vi "Read Image Metadata FIFO.vi"(0 "fpga inteface in":refnum<k20>, 5 "display channel number":i32, 7 "number of images":u32, 11 "error in (no error)":errorcluster) -> (4 "fpga interface out":refnum<k20>, 6 "image metadata":T1[](array[typedef]), 8 "images remaining":u32, 15 "error out":errorcluster)   [LabVIEW 2023, in "GettingStarted_Common_148X_Host.lvlib"]
uses:
  GettingStarted_Common_148X_Host.lvlib
  FPGA/Common/Types/Image Metadata.ctl
  <instrlib>/FlexRIO/CSI-2/v2/Common/Types/LLP Data Type.ctl
  Types/148x_Common_FPGA_Reference.ctl
  <vilib>/rvi/errors/niLvFpgaAdjustHostInterfaceError.vi
  <instrlib>/_niInstr/Data Formatting/v1/FPGA/Private/Convert/U64 array to Boolean Array.vi
  <vilib>/rvi/interface/nirviMethod/nirviMethod.xnode
  <vilib>/FPGAPlugInAG/Dynamic/niLvFpga_ReadFifo_Dynamic.vi
  <vilib>/rvi/errors/niLvFpgaMergeErrorWithErrorCode.vi
  <instrlib>/_niInstr/Data Formatting/v1/FPGA/niInstr Data Formatting v1 FPGA.lvlib
  <instrlib>/FlexRIO/CSI-2/v2/Common/NI CSI-2 API Common v2.lvlib
  FPGA/Common/GettingStarted_Common_148X_FPGA.lvlib
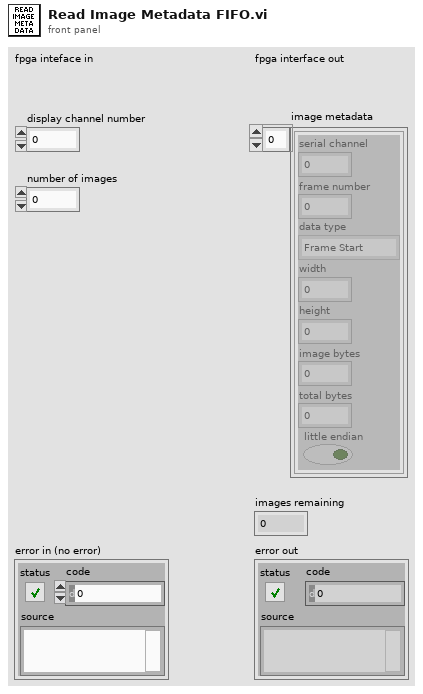
[diagram p1: front panel]
types:
  T1 = typedef "GettingStarted_Common_148X_FPGA.lvlib/Image Metadata.ctl" = cluster{"serial channel":fxp<+,3,3>, "frame number":u16, "data type":T2, "width":u16, "height":u16, "image bytes":u32, "total bytes":u32, "little endian":bool}
  T2 = typedef "NI CSI-2 API Common v2.lvlib/LLP Data Type.ctl" = enum8{"Frame Start", "Frame End", "Line Start", "Line End", "End of Transmission", "Reserved 0", "Reserved 1", "Reserved 2", "Generic Short Packet 1", "Generic Short Packet 2", "Generic Short Packet 3", "Generic Short Packet 4", "Generic Short Packet 5", "Generic Short Packet 6", "Generic Short Packet 7", "Generic Short Packet 8", "Null", "Blanking Data", "Embedded 8-bit non Image Data", "Generic Long Packet 1", "Generic Long Packet 2", "Generic Long Packet 3", "Generic Long Packet 4", "Reserved 3", "YUV420 8-bit", "YUV420 10-bit", "Legacy YUV420 8-bit", "Reserved 4", "YUV420 8-bit Chroma Shifted", "YUV420 10-bit Chroma Shifted", "YUV422 8-bit", "YUV422 10-bit", "RGB444", "RGB555", "RGB565", "RGB666", "RGB888", "Reserved 5", "Reserved 6", "RAW 24", "RAW 6", "RAW 7", "RAW 8", "RAW 10", "RAW 12", "RAW 14", "RAW 16", "RAW 20", "User Defined 8-bit Data 1", "User Defined 8-bit Data 2", "User Defined 8-bit Data 3", "User Defined 8-bit Data 4", "User Defined 8-bit Data 5", "User Defined 8-bit Data 6", "User Defined 8-bit Data 7", "User Defined 8-bit Data 8", "USL Command", "Reserved 7", "Reserved 8", "Reserved 9", "Reserved 10", "Reserved 11", "Reserved 12", "LRTE EPD Spacer"}
  T3 = typedef "GettingStarted_Common_148X_Host.lvlib/148x_Common_FPGA_Reference.ctl" = refnum<k20>
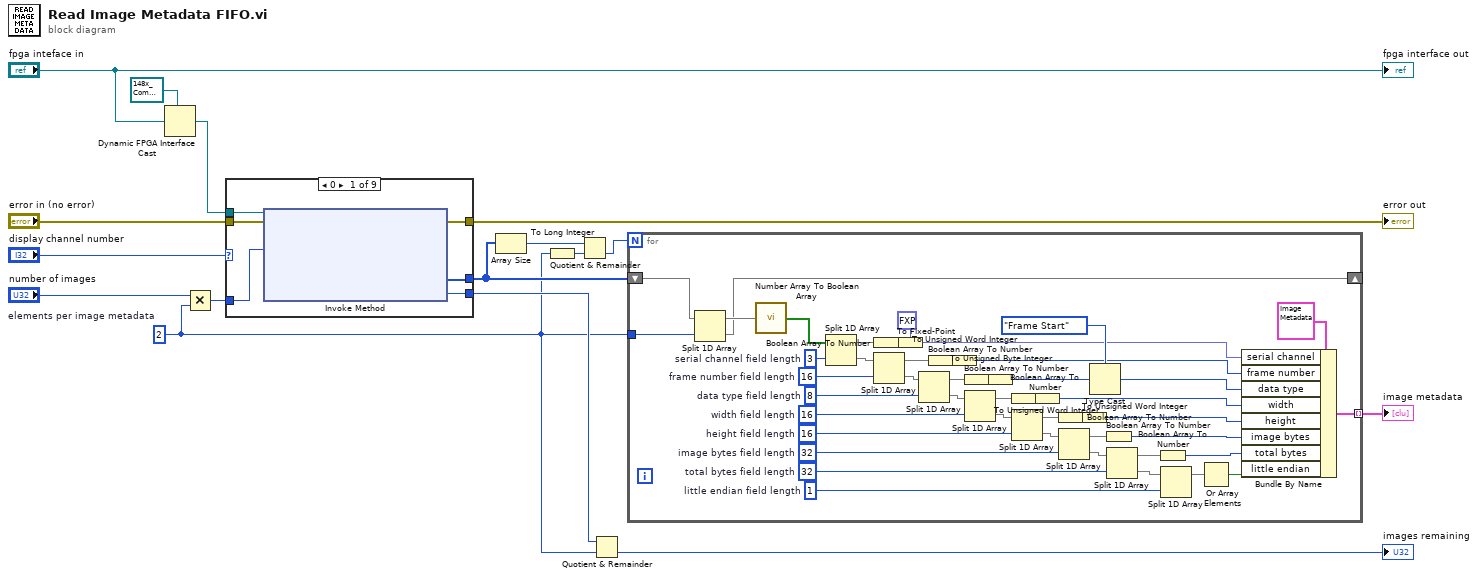
[diagram p0: block diagram]
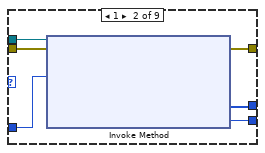
[diagram p2: hidden frame]
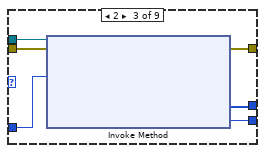
[diagram p3: hidden frame]
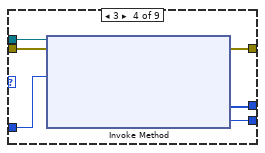
[diagram p4: hidden frame]
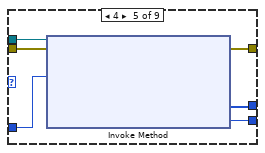
[diagram p5: hidden frame]
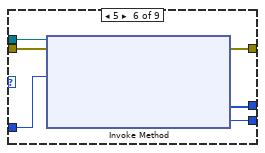
[diagram p6: hidden frame]
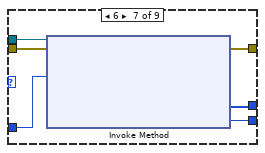
[diagram p7: hidden frame]
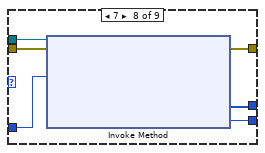
[diagram p8: hidden frame]
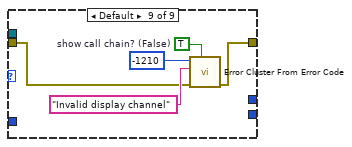
[diagram p9: hidden frame]
diagram:
  w3 = u32 2  # elements per image metadata
  n1 = Dynamic FPGA Interface Cast(Session In=T3 refnum ("FPGA VI Reference Out"), Type="fpga inteface in") -> (Session Out=w14:T3)
  n2 = Multiply(x="number of images", y=w3) -> (x*y=w9:u32)
  n3 = case shown="0" "display channel number" {
    tunnel: "error in (no error)" -> [w22 w28 w34 w40 w46 w52 w58 w64 w66]
    tunnel: w14 -> [w21 w27 w33 w39 w45 w51 w57 w63 _]
    tunnel: [w20 w26 w32 w38 w44 w50 w56 w62 w65] -> w10
    tunnel: w9 -> [w19 w25 w31 w37 w43 w49 w55 w61 _]
    tunnel: [w18 w24 w30 w36 w42 w48 w54 w60 _] -> w4
    tunnel: [w17 w23 w29 w35 w41 w47 w53 w59 _] -> w16
    frame 0 {
      n4 = xnode "Invoke Method"("FPGA VI Reference In"=w21, "error in"=w22, "Number of Elements"=w19) -> ("error out"=w20:errorcluster, "Data"=w18:u64[], "Elements Remaining"=w17:u32)  [unwired: 1 in, 1 out]
    }
    frame 1 {
      n5 = xnode "Invoke Method"("FPGA VI Reference In"=w27, "error in"=w28, "Number of Elements"=w25) -> ("error out"=w26:errorcluster, "Data"=w24:u64[], "Elements Remaining"=w23:u32)  [unwired: 1 in, 1 out]
    }
    frame 2 {
      n6 = xnode "Invoke Method"("FPGA VI Reference In"=w33, "error in"=w34, "Number of Elements"=w31) -> ("error out"=w32:errorcluster, "Data"=w30:u64[], "Elements Remaining"=w29:u32)  [unwired: 1 in, 1 out]
    }
    frame 3 {
      n7 = xnode "Invoke Method"("FPGA VI Reference In"=w39, "error in"=w40, "Number of Elements"=w37) -> ("error out"=w38:errorcluster, "Data"=w36:u64[], "Elements Remaining"=w35:u32)  [unwired: 1 in, 1 out]
    }
    frame 4 {
      n8 = xnode "Invoke Method"("FPGA VI Reference In"=w45, "error in"=w46, "Number of Elements"=w43) -> ("error out"=w44:errorcluster, "Data"=w42:u64[], "Elements Remaining"=w41:u32)  [unwired: 1 in, 1 out]
    }
    frame 5 {
      n9 = xnode "Invoke Method"("FPGA VI Reference In"=w51, "error in"=w52, "Number of Elements"=w49) -> ("error out"=w50:errorcluster, "Data"=w48:u64[], "Elements Remaining"=w47:u32)  [unwired: 1 in, 1 out]
    }
    frame 6 {
      n10 = xnode "Invoke Method"("FPGA VI Reference In"=w57, "error in"=w58, "Number of Elements"=w55) -> ("error out"=w56:errorcluster, "Data"=w54:u64[], "Elements Remaining"=w53:u32)  [unwired: 1 in, 1 out]
    }
    frame 7 {
      n11 = xnode "Invoke Method"("FPGA VI Reference In"=w63, "error in"=w64, "Number of Elements"=w61) -> ("error out"=w62:errorcluster, "Data"=w60:u64[], "Elements Remaining"=w59:u32)  [unwired: 1 in, 1 out]
    }
    frame Default {
      w67 = TRUE  # show call chain? (False)
      n12 = call <vilib>:"Error Cluster From Error Code.vi"("show call chain? (False)"=w67, "error in (no error)"=w66, "error message (\"\")"="Invalid display channel" ("error message (\"\")"), "error code (0)"=-1210) -> ("error out"=w65:errorcluster)  [unwired: 5 in]
    }
  }
  "error out" <- w10
  n13 = Array Size(array=w4) -> (size(s)=w5:i32)
  n14 = To Long Integer(number=w3) -> (32bit integer=w1:i32)
  n15 = Quotient & Remainder(x=w5, y=w1) -> (floor(x/y)=w2:i32)  [unwired: 1 out]
  n16 = Quotient & Remainder(x=w16, y=w3) -> (floor(x/y)=→"images remaining":u32)  [unwired: 1 out]
  n17 = for {
    N: w2 -> [_]
    shift-right: [w86] -> _
    shift-left: w4 -> [w115]
    tunnel: w3 -> [w114]
    tunnel: [w87] -> w8 mode=indexing
    w76 = 16  # frame number field length
    w81 = 1  # little endian field length
    w103 = 32  # total bytes field length
    w105 = 32  # image bytes field length
    w107 = 16  # height field length
    w109 = 16  # width field length
    w77 = 8  # data type field length
    w111 = 3  # serial channel field length
    n18 = Split 1D Array(array=w115, index=w114) -> (first subarray=w113:u64[], second subarray=w86:u64[])
    n19 = call-poly <instrlib>:"Number Array To Boolean Array.vi"("data in"=w113) -> ("data out"=w112:bool[])  [unwired: 14 in]
    n20 = Split 1D Array(array=w112, index=w111) -> (first subarray=w91:bool[], second subarray=w110:bool[])
    n21 = Boolean Array To Number(Boolean array=w91) -> (number=w92:u32)
    n22 = Split 1D Array(array=w110, index=w76) -> (first subarray=w72:bool[], second subarray=w79:bool[])
    n23 = To Fixed-Point(fixed-point type=fxp<+,3,3> 0.0, number=w92) -> (fixed-point=w80:fxp<+,3,3>)
    n24 = Split 1D Array(array=w79, index=w77) -> (first subarray=w73:bool[], second subarray=w78:bool[])
    n25 = Boolean Array To Number(Boolean array=w72) -> (number=w71:u32)
    n26 = To Unsigned Word Integer(number=w71) -> (unsigned 16bit integer=w70:u16)
    n27 = Boolean Array To Number(Boolean array=w73) -> (number=w90:u32)
    n28 = Split 1D Array(array=w78, index=w109) -> (first subarray=w94:bool[], second subarray=w108:bool[])
    n29 = To Unsigned Byte Integer(number=w90) -> (unsigned 8bit integer=w89:u8)
    n30 = Boolean Array To Number(Boolean array=w94) -> (number=w95:u32)
    n31 = Split 1D Array(array=w108, index=w107) -> (first subarray=w98:bool[], second subarray=w106:bool[])
    n32 = To Unsigned Word Integer(number=w95) -> (unsigned 16bit integer=w93:u16)
    n33 = Boolean Array To Number(Boolean array=w98) -> (number=w97:u32)
    n34 = Split 1D Array(array=w106, index=w105) -> (first subarray=w100:bool[], second subarray=w104:bool[])
    n35 = To Unsigned Word Integer(number=w97) -> (unsigned 16bit integer=w96:u16)
    n36 = Type Cast(type=LLP_Data_Type."Frame Start" ("data type"), x=w89) -> (*(type *) &x=w74:T2)
    n37 = Boolean Array To Number(Boolean array=w100) -> (number=w99:u32)
    n38 = Split 1D Array(array=w104, index=w103) -> (first subarray=w83:bool[], second subarray=w84:bool[])
    n39 = Boolean Array To Number(Boolean array=w83) -> (number=w82:u32)
    n40 = Split 1D Array(array=w84, index=w81) -> (first subarray=w85:bool[])  [unwired: 1 out]
    n41 = Or Array Elements(Boolean array=w85) -> (logical OR=w101:bool)
    n42 = Bundle By Name(cluster=T1 {"serial channel"=0.0, "frame number"=0, "data type"=enum."Frame Start", "width"=0, "height"=0, "image bytes"=0, "total bytes"=0, "little endian"=FALSE} ("image metadata"), "serial channel"=w80, "frame number"=w70, "data type"=w74, "width"=w93, "height"=w96, "image bytes"=w99, "total bytes"=w82, "little endian"=w101) -> (w87:T1)
  }
  "image metadata" <- w8
  "fpga interface out" <- "fpga inteface in"
